vi "FestoCPX.Station.Emg.Wait.Edge.vi"(6 "timeout [ms] (1000)":u32=1000, 8 "error in":errorcluster, 10 "Position":T2) -> (0 "error out":errorcluster, 3 "timeout":bool)   [LabVIEW 2015]
uses:
  Station/Station.ValvePosition.ctl
  FestoCPX.Station.EmgState.ctl
panel:
  out "safety":T1
  out "delay":u32
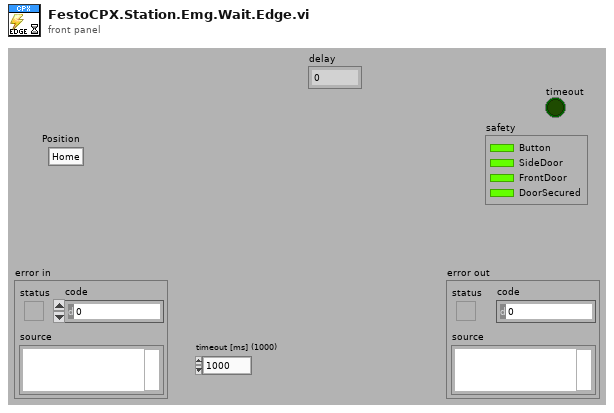
[diagram p1: front panel]
types:
  T1 = typedef "FestoCPX.Station.EmgState.ctl" = cluster{"Button":bool, "SideDoor":bool, "FrontDoor":bool, "DoorSecured":bool}
  T2 = typedef "Station.ValvePosition.ctl" = enum16{"Home", "Work"}
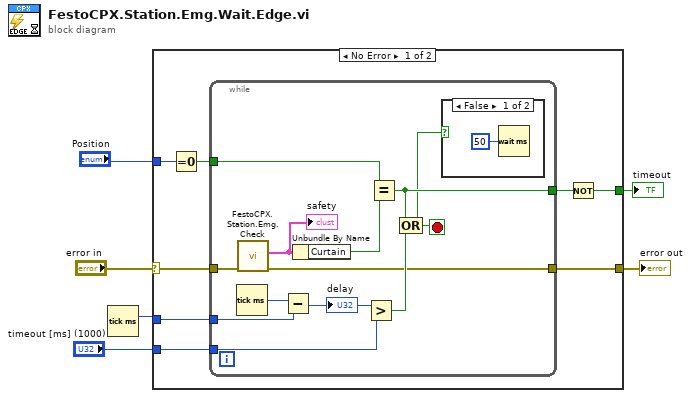
[diagram p0: block diagram]
diagram:
  n1 = Tick Count (ms)() -> (millisecond timer value=w2:u32)
  n2 = case shown="No Error" "error in" {
    selector: "error in" -> [w14 w28]
    tunnel: [w10 w28] -> w6
    tunnel: "Position" -> [w13 _]
    tunnel: w2 -> [w12 _]
    tunnel: [w7 _] -> w3
    tunnel: "timeout [ms] (1000)" -> [w8 _]
    frame No Error {
      n3 = Equal To 0?(x=w13) -> (x = 0?=w11:bool)
      n4 = while {
        tunnel: w14 -> [w20]
        tunnel: [w18] -> w10
        tunnel: w11 -> [w26]
        tunnel: w12 -> [w23]
        tunnel: [w17] -> w9
        tunnel: w8 -> [w22]
        stop <- w16 stop-if-true
        n5 = Tick Count (ms)() -> (millisecond timer value=w24:u32)
        n6 = call "FestoCPX.Station.Emg.Check.vi"("error in"=w20) -> ("error out"=w18:errorcluster, "Emg"=w15:T1)  [unwired: 8 in, 1 out]
        "safety" <- w15
        n7 = Subtract(x=w24, y=w23) -> (x-y=w21:u32)
        "delay" <- w21
        n8 = Unbundle By Name(w15) -> ("Curtain"=w19:bool)
        n9 = Greater?(x=w21, y=w22) -> (0:w25:bool)
        n10 = Equal?(x=w26, y=w19) -> (x = y?=w17:bool)
        n11 = Compound Arithmetic op=OR(w17, w25) -> (w16:bool)
        n12 = case shown="False" w16 {
          frame False {
            n13 = Wait (ms)(milliseconds to wait=u32 50) -> ()  [unwired: 1 out]
          }
          frame True {
          }
        }
      }
      n14 = Not(x=w9) -> (.not. x?=w7:bool)
    }
    frame Error {
    }
  }
  "error out" <- w6
  "timeout" <- w3
